vi "Page_Exclusions_Initialize.vi"(8 "error in (no error)":errorcluster, 9 "ctlReferences":T1, 11 "AB_SourceDistribution in":refnum<class "AB_SourceDistribution.lvclass">) -> (0 "error out":errorcluster, 3 "AB_SourceDistribution out":refnum<class "AB_SourceDistribution.lvclass">)   [LabVIEW 2020, in "AB_SourceDistribution.lvclass"]
uses:
  <vilib>/AppBuilder/AB_Classes/SourceDistribution/AB_SourceDistribution.lvclass
  <resource>/Framework/Providers/Builds/AppBuilder/AB_UI_Page_Exclusions_References.ctl
  <vilib>/AppBuilder/AB_Classes/Build/AB_Build.lvclass
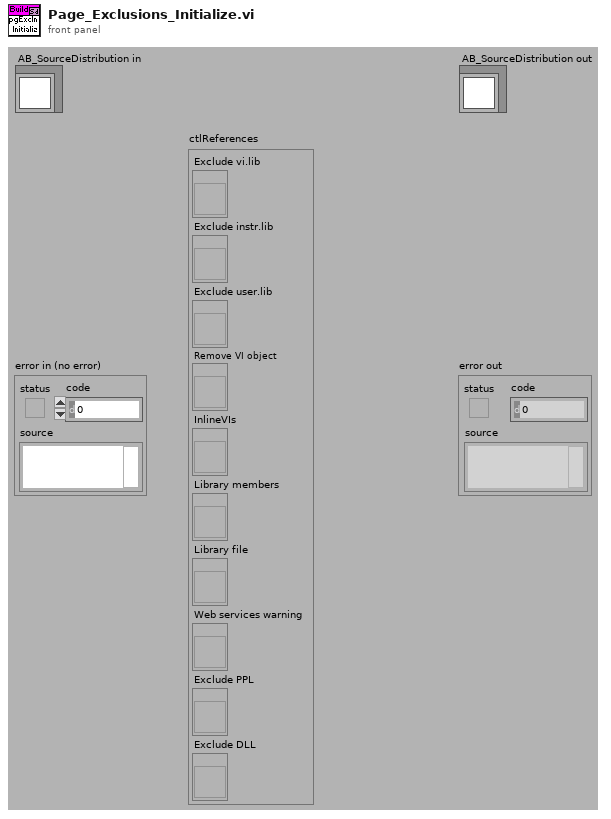
[diagram p1: front panel]
types:
  T1 = typedef "AB_UI_Page_Exclusions_References.ctl" = cluster{"Exclude vi.lib":refnum<vi>, "Exclude instr.lib":refnum<vi>, "Exclude user.lib":refnum<vi>, "Remove VI object":refnum<vi>, "InlineVIs":refnum<vi>, "Library members":refnum<vi>, "Library file":refnum<vi>, "Web services warning":refnum<vi>, "Exclude PPL":refnum<vi>, "Exclude DLL":refnum<vi>}
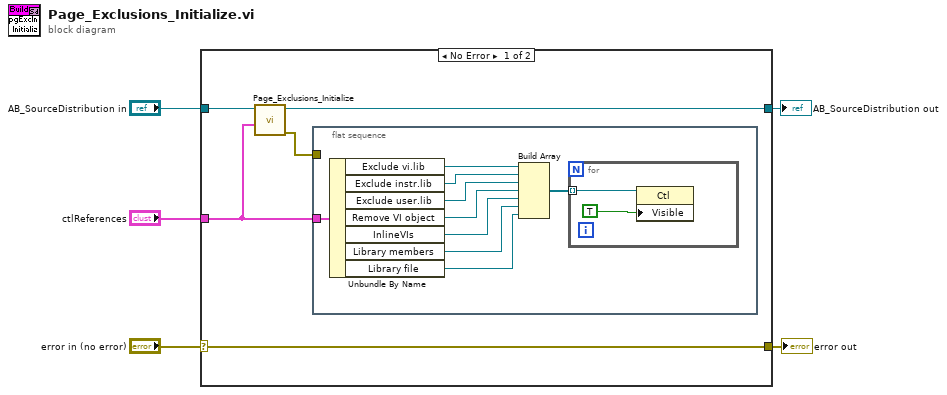
[diagram p0: block diagram]
diagram:
  n1 = case shown="No Error" "error in (no error)" {
    selector: "error in (no error)" -> [w10 w23]
    tunnel: [w10 w23] -> w4
    tunnel: [w8 w22] -> w2
    tunnel: "AB_SourceDistribution in" -> [w9 w22]
    tunnel: "ctlReferences" -> [w7 _]
    frame No Error {
      n2 = call-parent "Page_Exclusions_Initialize.vi"("ctlReferences"=w7, "AB_Build in"=w9) -> ("error out"=w6:errorcluster, "AB_Build out"=w8:refnum<class "AB_SourceDistribution.lvclass">)  [unwired: 8 in]
      n3 = flat-sequence {
        tunnel: w7 -> [w19]
        tunnel: w6 -> [_]
        frame #0 {
          n4 = Unbundle By Name(w19) -> ("Exclude vi.lib"=w18:refnum<vi>, "Exclude instr.lib"=w17:refnum<vi>, "Exclude user.lib"=w16:refnum<vi>, "Remove VI object"=w15:refnum<vi>, "InlineVIs"=w13:refnum<vi>, "Library members"=w12:refnum<vi>, "Library file"=w11:refnum<vi>)
          n5 = Build Array(w18, w17, w16, w15, w13, w12, w11) -> (w14:refnum<vi>[])
          n6 = for {
            tunnel: w14 -> [w21] mode=indexing
            n7 = property class="Ctl"(reference=w21, "Visible"=TRUE) -> ()  [unwired: 1 in, 2 out]
          }
        }
      }
    }
    frame Error {
    }
  }
  "error out" <- w4
  "AB_SourceDistribution out" <- w2
